vi "Find Unexpected Deps.vi"() -> ()   [LabVIEW 2019, in "DepsWatchToolsMenu.lvlib"]
doc: "GUI to compare LabVIEW code between currently checked out branch with any other branch or any of its commits.\n\n(c) 2024 Soliton Technologies. All rights reserved."
uses:
  DepsWatchToolsMenu.lvlib
  vi.lib/DepsWatch/Typedefs/DepsCheckResult.ctl
  <vilib>/Hampel Software Engineering/Git API/Git API/GIT-api.lvclass
  <vilib>/Hampel Software Engineering/Git API/Git API/GIT-api.lvclass/GIT-api.ctl
  <vilib>/Hampel Software Engineering/Git API/Git API/Controls/GIT-Repository States.ctl
  <vilib>/Hampel Software Engineering/Git API/Git API/Accessors/GIT-Set Working Dir.vi
  <userlib>/_OpenG.lib/file/file.llb/Valid Path - Traditional__ogtk.vi
  <userlib>/_OpenG.lib/file/file.llb/File Exists - Scalar__ogtk.vi
  vi.lib/DepsWatch/DepsWatch.lvlib
panel:
  in  "Tab Control":T1(tab)=enum."Main UI"
  in  "Check Changed Libraries Only?":bool
  out "Unexpected / Missing Deps":T2[](array[typedef])
  in  "Branch to Compare":string(combo)="origin/main"
  in  "Refresh Current Branch":bool
  out "Current Branch":string="origin/main" caption="Current Compare"
  out "Current Branch Status":string
  in  "Stop":bool
  in  "Repository Path":path
  in  "Compare":bool
  # "1. Checkout the branch of interest in your system using any method - Git command line, Desktop Git GUI Clients etc.,\n\n2. Specify the local Repository Path.\n\n3. Verify the current branch, its status and select a branch or commit based on the Compare Mode and click on Compare to display the file changes.\n\n4. Double click on a file to initiate LabVIEW code comparison.\n\n5. Once done with required comparisons, exit the tool by closing the window. The tool cleans up the temporary files added during comparison.\n\n\nNote:\n1. This tool uses LabVIEW's VI Comparison Tool which requires LabVIEW Professional Development System.\n2. It is recommended to not use other Git Clients actively when comparing files using this tool to avoid Git command related errors.\n3. It is recommended to commit all changes (working copy) before using this tool for comparison."
  # "This tool uses git diff command to identify the changes. Hence it is recommended to commit all the changes (working copy) to have them considered for comparison. For code comparison, this tool uses LabVIEW's built in VI Comparison Tool.\n\nExample: Identify changes in current branch when comparing with other branch\n\n---A---B---C---D    <== other branch\n               \\\n                 E---F      <== current branch\n\n1. We will need to identify only the file changes introduced by current branch. E and F commits are those changes in the above example (commits after the common ancestor B).\n2. For the identified file changes compare with the other branch (D) to see how it differs. These differences will be our current branch changelist.\n\nWhy only current branch changes?\nIt is most useful to see how the current branch will modify the files when it is getting merged. Best use case for displaying only current branch changelist will be for Pull Request reviews."
  # "1. Repository Path - Local repository path (the top level folder with '.git' hidden folder in it). Git API will be initialized for this repository.\n\n2. Current Branch - Currently checked out branch. The status of the current branch is also displayed at top right. Click Refresh button to update the current branch if it is changed in the system or received new changes via Git Pull.\n\n3. Compare Mode - Select the type of comparison. You can compare the current branch with another branch or with a particular commit of a selected branch.\n\nIn branch comparison mode, you can enter the branch name for comparison in Branch to Compare. Remote branches usually start with \"origin/\" and local branches do not have \"origin/\" prefix. The branch's recent commit is displayed in Recent Commit and its details in Commit Details for reference. \n\nIn commit comparison mode, the commits available in the branch selected in Select Branch are listed in Commit to Compare. For the commit selected in Commit to Compare, its details will be displayed in the Commit Details. Use Commits to Fetch to limit the number of commits obtained and improve the loading time.\n\n     Note: Git doesn't maintain information on when the branch is created. So, all the commits of the selected branch will be displayed (all the way up to the very first commit after repository creation). Without a limit, it increases loading time.\n\n4. Compare - Identifies the file changes and Current Branch Changelist table shows the list of all files that are different in the current branch compared to the branch/commit selected.\n\n     Note: The other branch/commit in comparison would have introduced its own changes that are not part of current branch. Those changes will not be displayed.\n\n5. Filter LabVIEW VI and Control Files - Filter files except VI and CTL files. These require LabVIEW to compare but project, library and classes are text files that can be easily reviewed in the desktop Git GUI clients or in Pull Request of Git web services.\n\n6. LabVIEW Compare Options - Options to decide what to compare in the code. Set the required options before initiating code compare.\n\n7. Double click on the file you wish to compare. LabVIEW opens the compare window for the file from the current branch and the file from the other branch/commit (file will be suffixed with TEMP). It may take a while if the VI/CTL have lot of dependencies to load. Having the project pre-opened and opening this tool from that instance may reduce the loading time. Note that the file from the other branch/commit in comparison may be missing its dependent files which may not be available in the current branch or deleted in the current branch commits. This will cause the file to be in a broken state but does not affect the comparison. Another reason for the broken state may be due to the parent library/class not recognizing this new file with the suffix but this as well will not affect the comparison.\n\n     Note: The files from other branch/commit are placed at the same location in the current branch so that the LabVIEW can load the dependencies appropriately.\n\n8. Viewed Status (mixed checkbox) - A tick mark appears for every file compared or opened. Use the mixed checkbox (below the Current Branch Changelist) to control status for all files.\n\n     Note: Viewed status is only a visual aid for tracking and does not have any other function other than that.\n\n9. Panel Close - Stops the tools execution after removing all the new files introduced into the current branch (TEMP files)."
  # "This GUI helps identify unexpected dependencies across all libraries in a repository. It also supports branch-to-branch comparison, allowing users to analyze dependency changes between any two branches and validate dependencies only for the modified libraries."
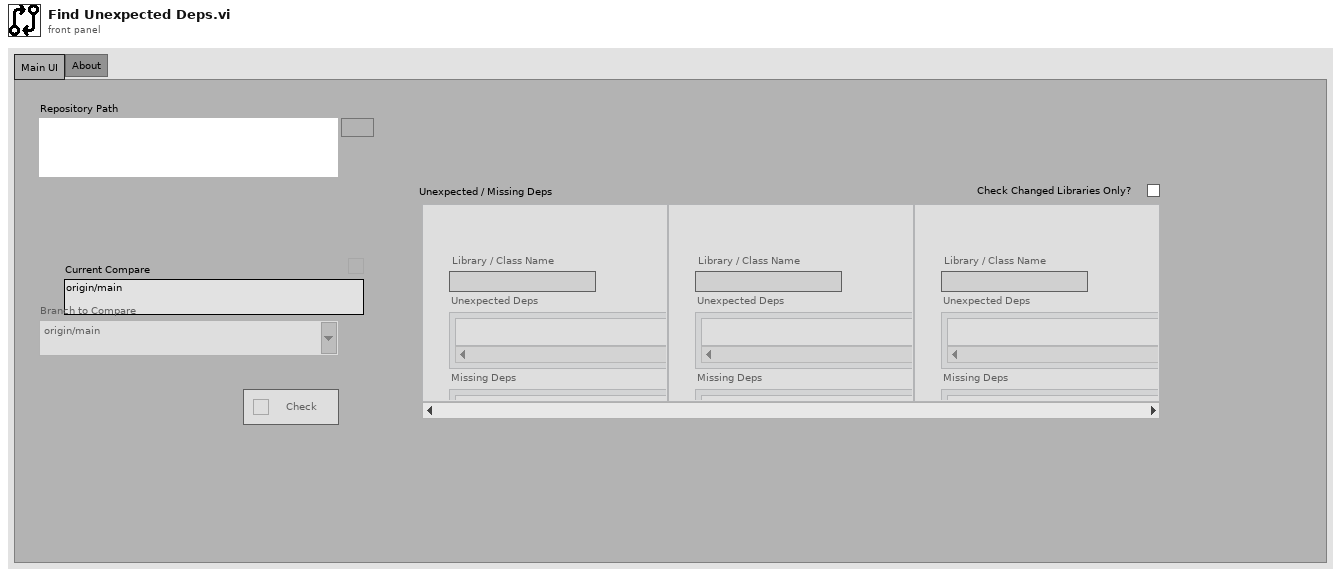
[diagram p1: front panel]
types:
  T1 = enum32{"Getting Started", "How it Works?", "Main UI", "Help", "About"}
  T2 = typedef "DepsWatch.lvlib/DepsCheckResult.ctl" = cluster{"Library / Class Name":string, "Unexpected Deps":cluster{"Dependency":string, "IsDirect?":bool}[], "Missing Deps":cluster{"Dependency":string, "IsDirect?":bool}[]}
  T3 = cluster{"Repository Path":path, "Git API Object":refnum<class "GIT-api.lvclass">, "Git API Initialized?":bool, "Current Branch":string, "Branch to Compare":string, "Check Changed Libraries Only?":bool, "Failures":T2[]}
  T4 = typedef "GIT-API-for-LabVIEW.lvlib/GIT-api.lvclass/GIT-Repository States.ctl" = enum16{"up-to-date", "behind", "ahead", "diverged", "unpublished", "detached", "unknown"}
  T5 = enum8{"Enabled", "Disabled", "Disabled and Grayed Out"}
  T6 = typedef "DepsWatch.lvlib/CICDPathConfigs.ctl" = cluster{"GlobalIncludePaths":path[], "GlobalExcludePaths":path[], "BuildSpecsIncludePaths":path[], "ActualDepsIncludePaths":path[], "WorkspacePath":path, "SourceFolderPaths":path[], "ChangedFilesLogpaths":map{string, path}}
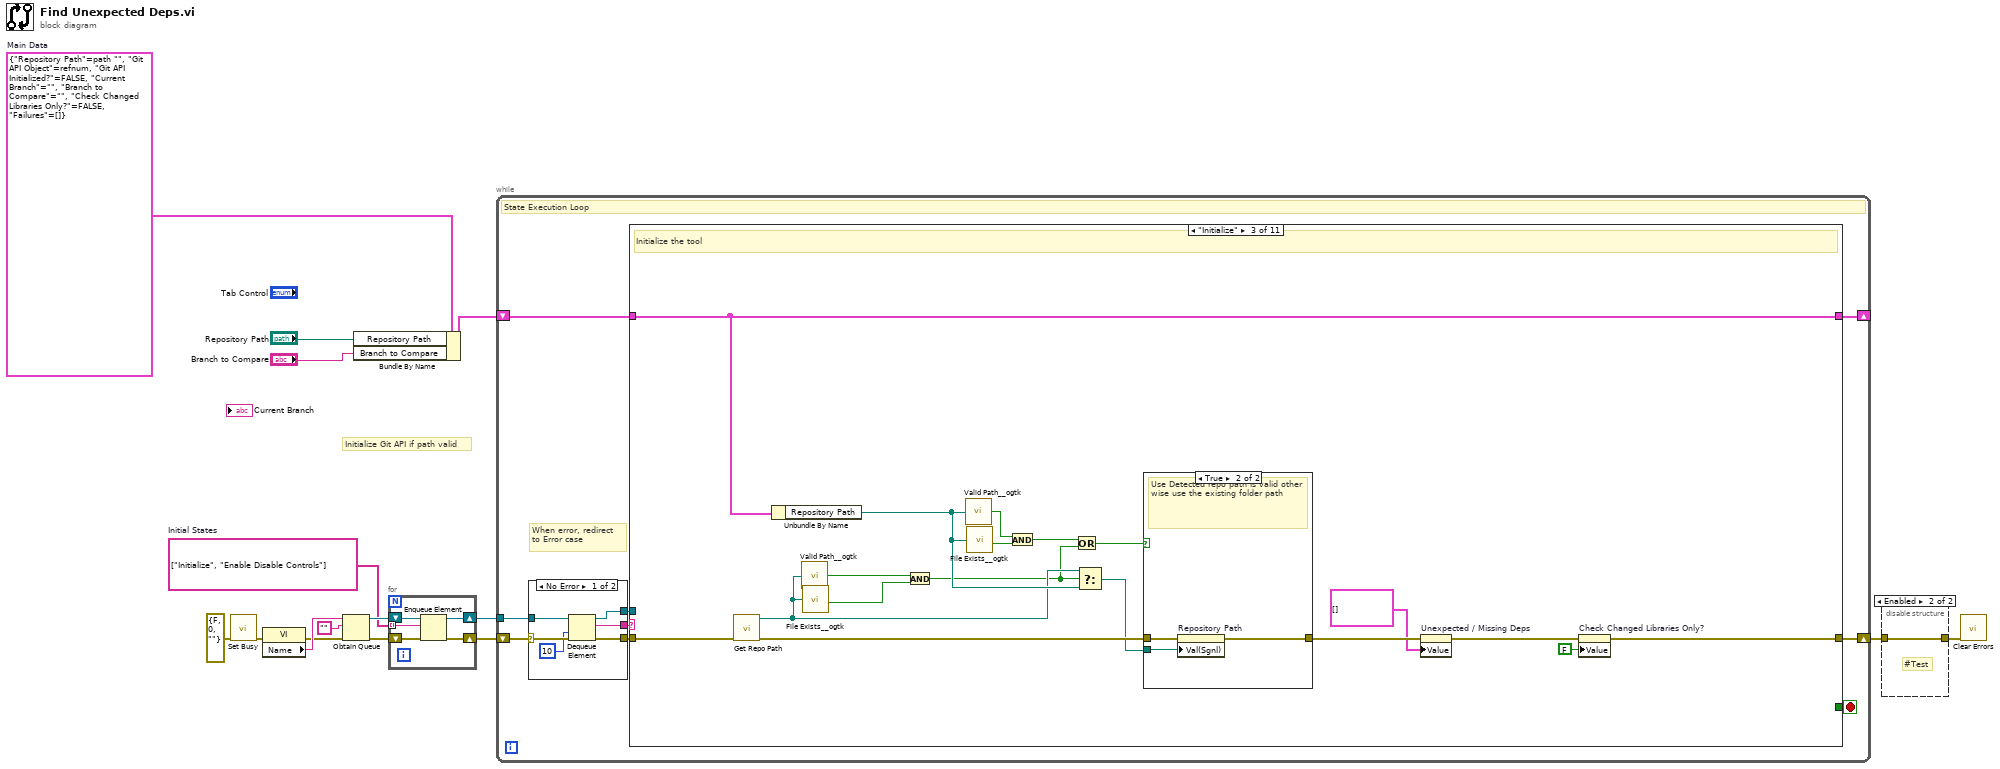
[diagram p0: block diagram]
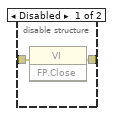
[diagram p2: hidden frame]
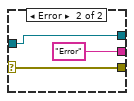
[diagram p3: hidden frame]
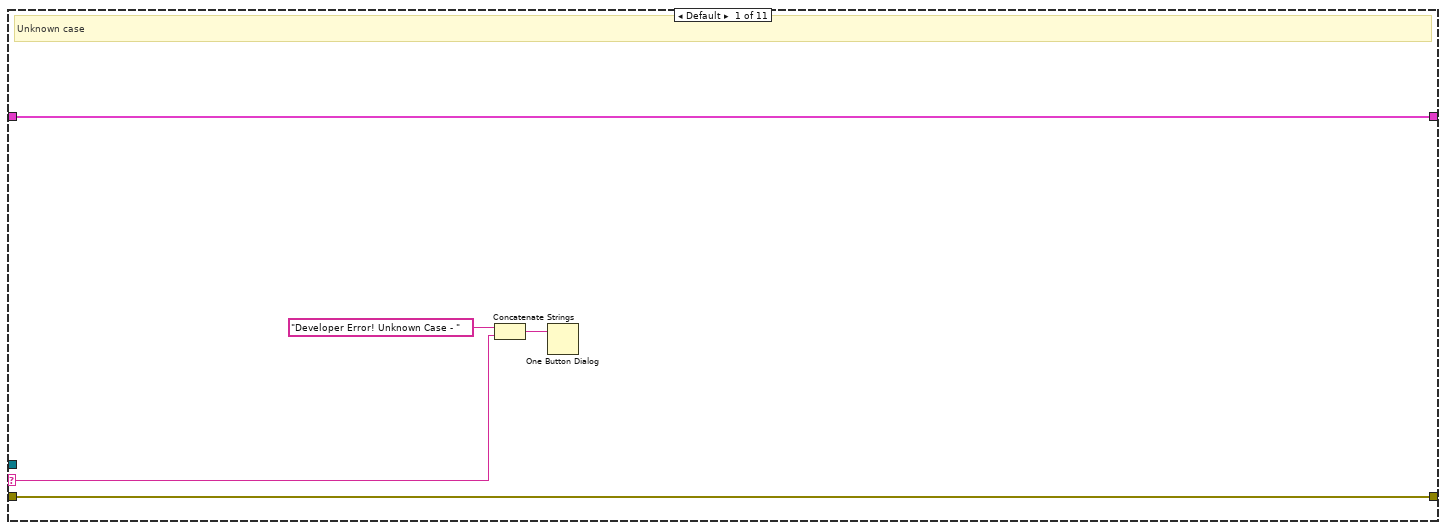
[diagram p4: hidden frame]
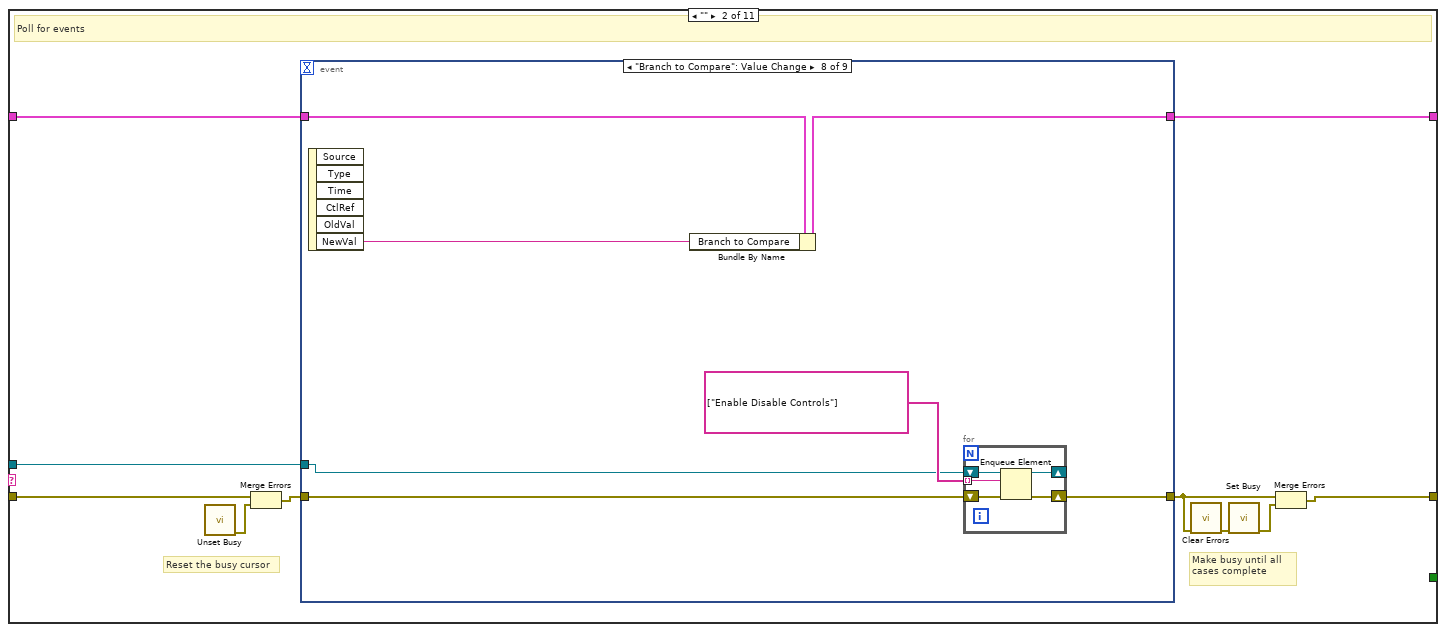
[diagram p5: hidden frame]
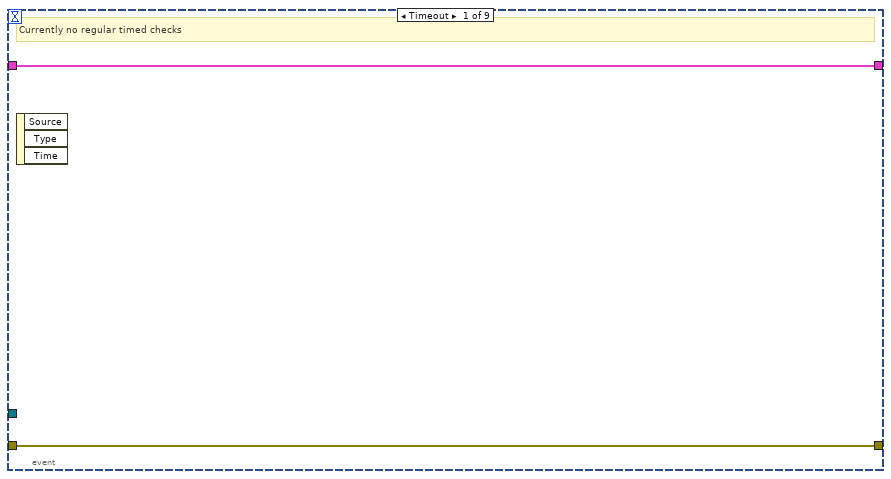
[diagram p6: hidden frame]
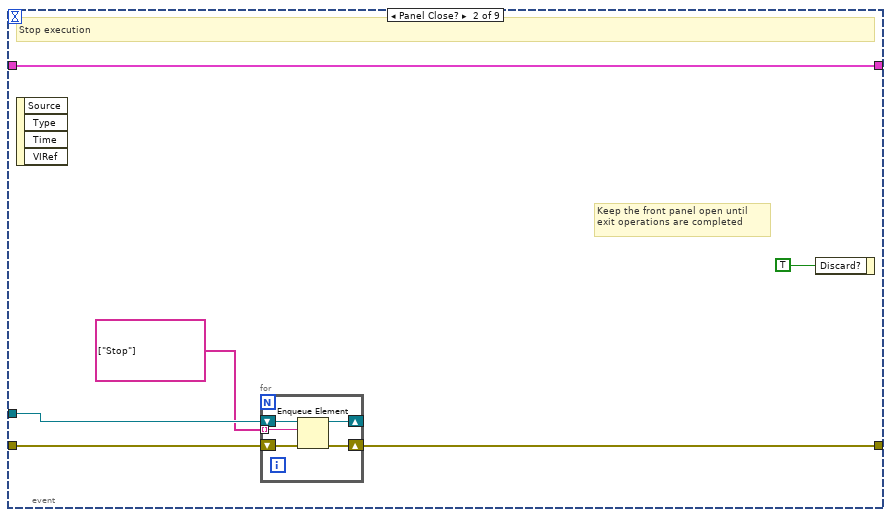
[diagram p7: hidden frame]
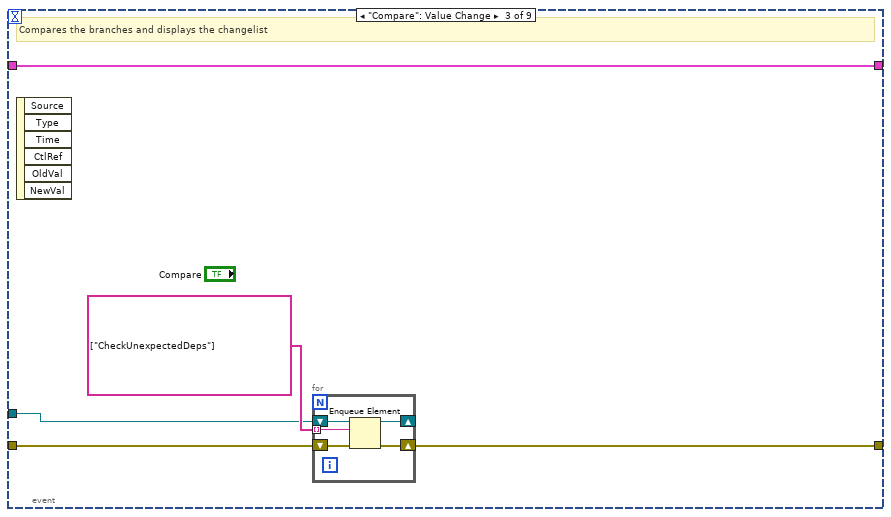
[diagram p8: hidden frame]
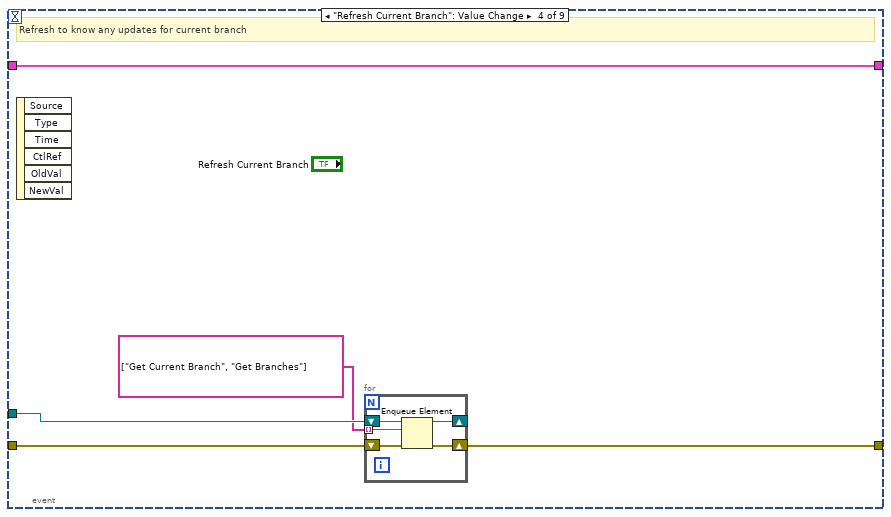
[diagram p9: hidden frame]
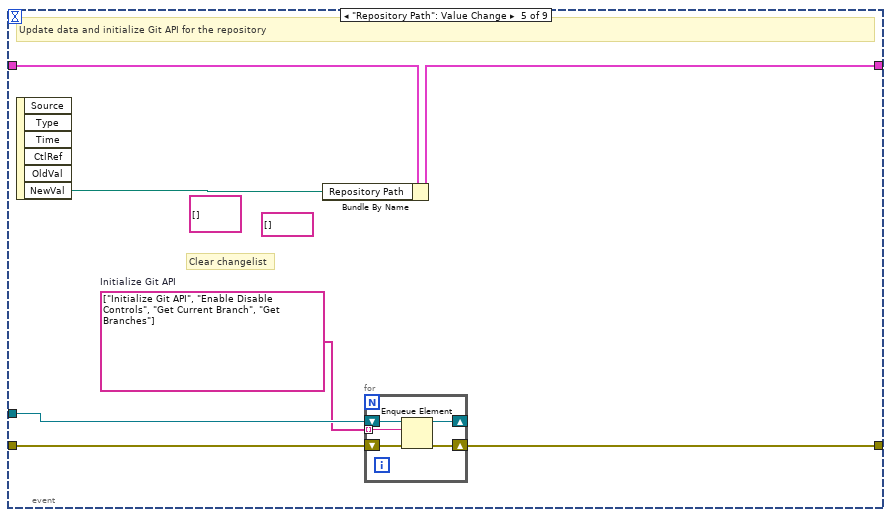
[diagram p10: hidden frame]
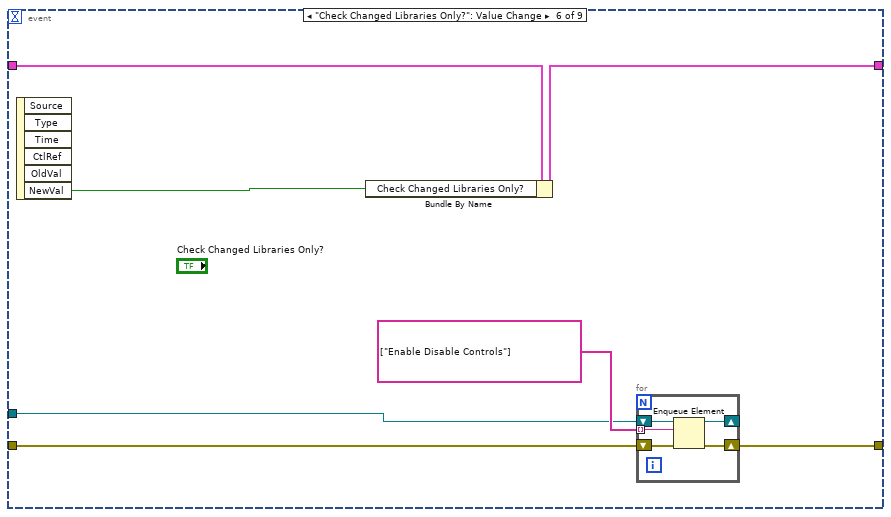
[diagram p11: hidden frame]
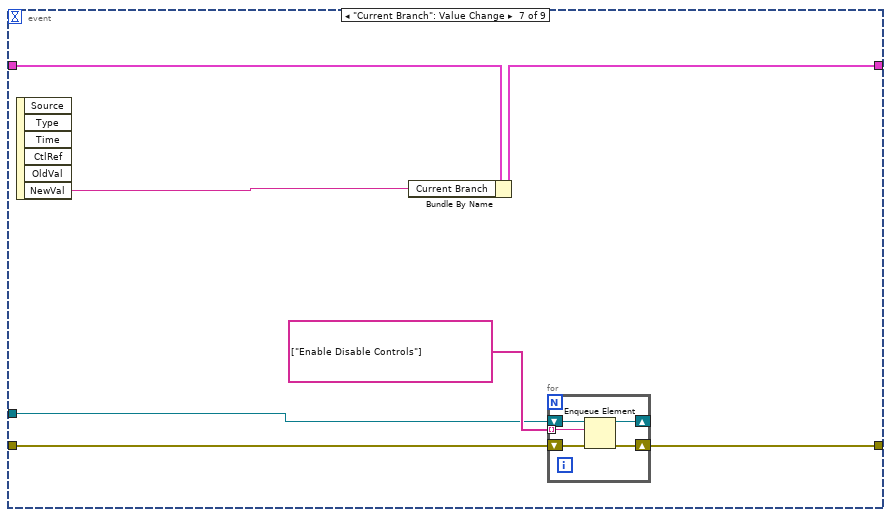
[diagram p12: hidden frame]
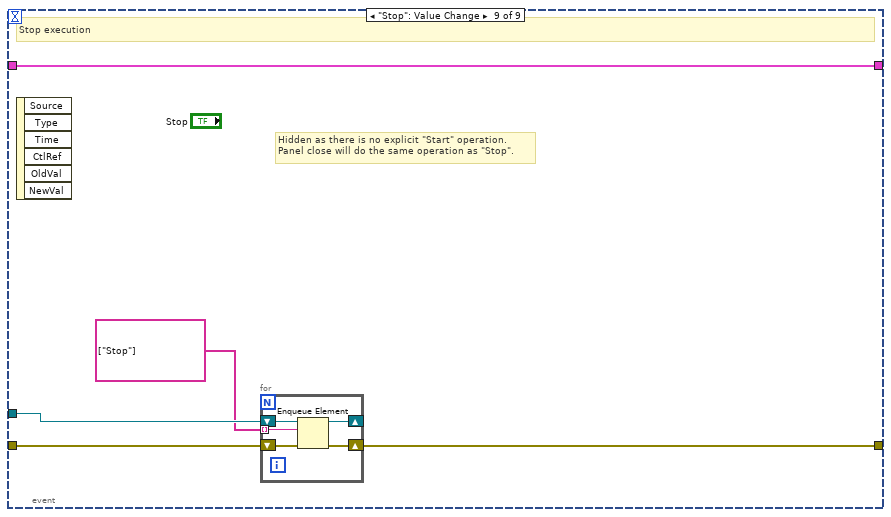
[diagram p13: hidden frame]
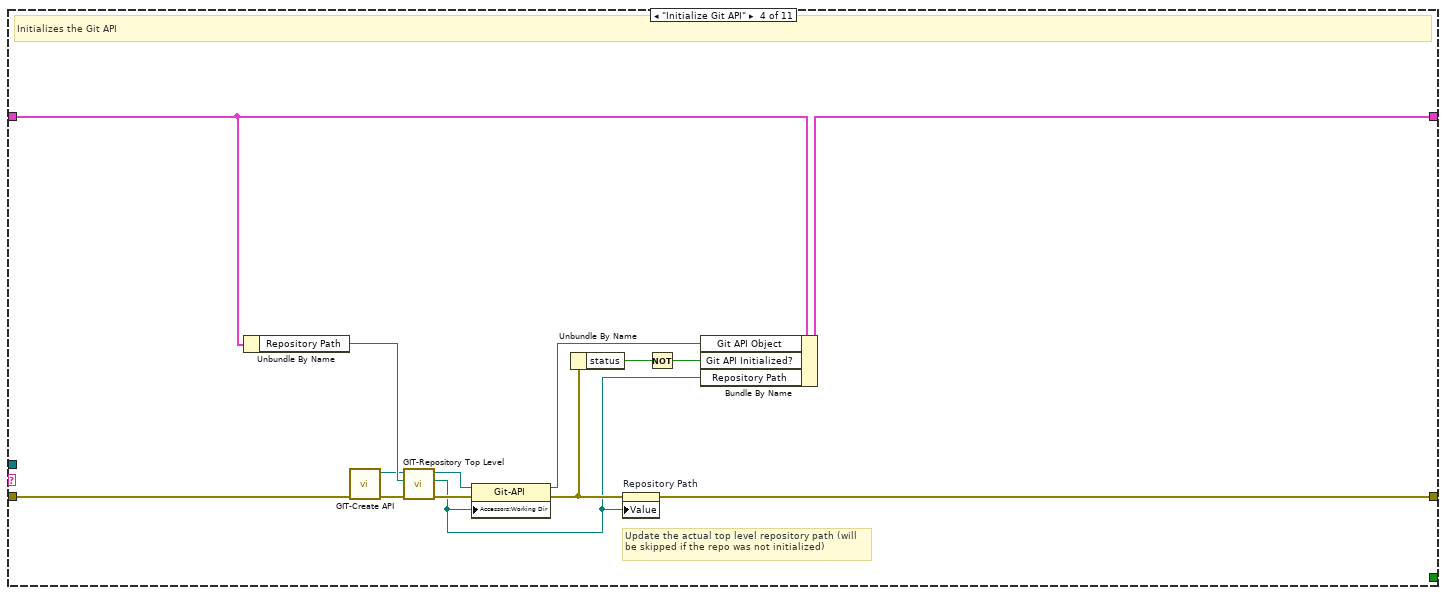
[diagram p15: hidden frame]
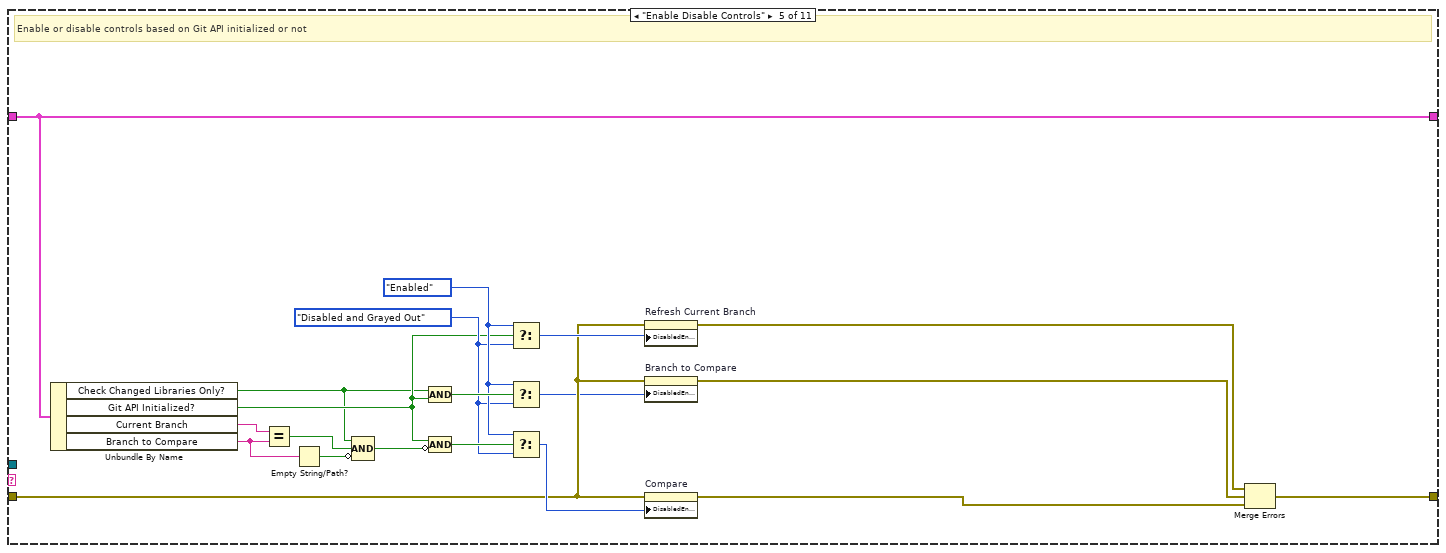
[diagram p16: hidden frame]
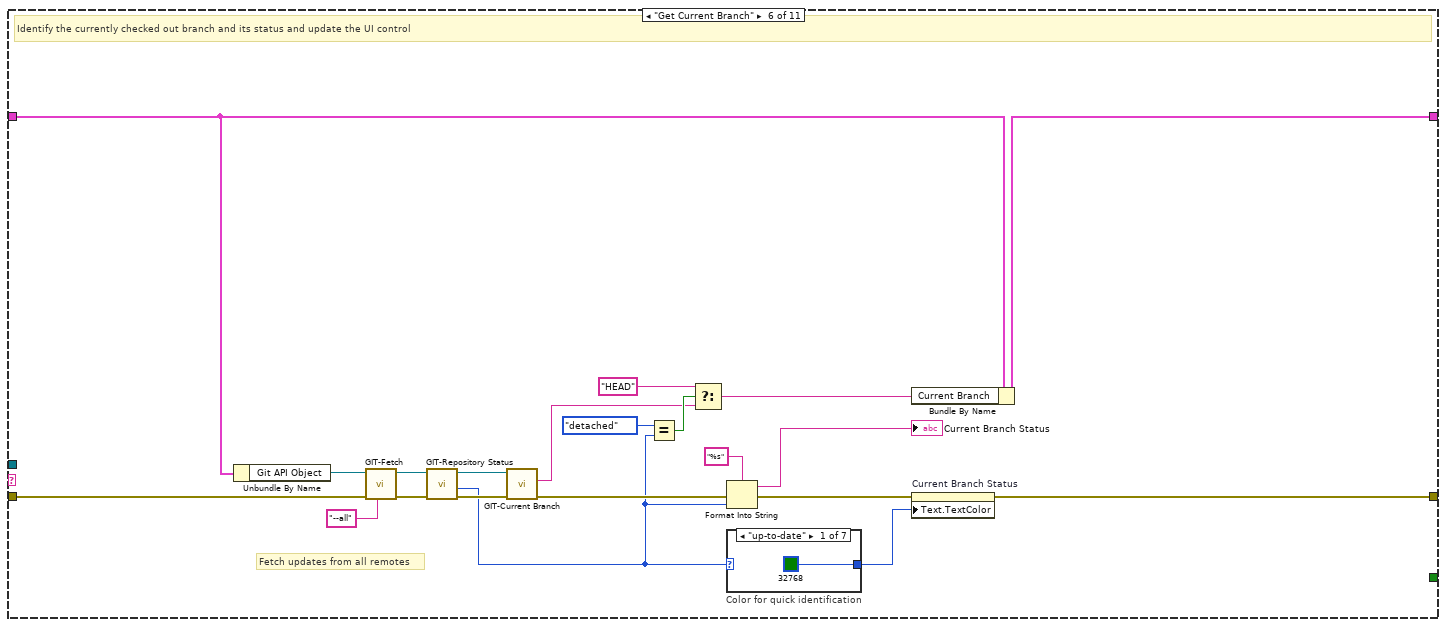
[diagram p17: hidden frame]
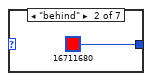
[diagram p18: hidden frame]
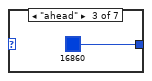
[diagram p19: hidden frame]
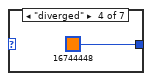
[diagram p20: hidden frame]
diagram:
  w1 = string[] ["Initialize", "Enable Disable Controls"]  # Initial States
  w13 = T3 {"Repository Path"=path "", "Git API Object"=refnum, "Git API Initialized?"=FALSE, "Current Branch"="", "Branch to Compare"="", "Check Changed Libraries Only?"=FALSE, "Failures"=[]}  # Main Data
  # "Initialize Git API if path valid"
  n1 = call <vilib>:"Set Busy.vi"("error in (no error)"=errorcluster {"status"=FALSE, "code"=0, "source"=""}) -> ("error out"=w6:errorcluster)  [unwired: 9 in, 1 out]
  n2 = property class="VI"(error in=w6) -> (error out=w15:errorcluster, "Name"=w16:string)  [unwired: 1 in, 1 out]
  n3 = Obtain Queue(name (unnamed)=w16, element data type="", error in (no error)=w15) -> (queue out=w11:refnum<queue>, error out=w8:errorcluster)  [unwired: 2 in, 1 out]
  n4 = Bundle By Name(cluster=w13, "Repository Path"="Repository Path", "Branch to Compare"="Branch to Compare") -> (w12:T3)
  n5 = for {
    tunnel: w1 -> [w18] mode=indexing
    shift-right: [w20] -> w10
    shift-left: w8 -> [w21]
    shift-right: [w17] -> w9
    shift-left: w11 -> [w19]
    n6 = Enqueue Element(queue=w19, element=w18, error in (no error)=w21) -> (queue out=w17:refnum<queue>, error out=w20:errorcluster)  [unwired: 1 in, 1 out]
  }
  n7 = while {
    shift-right: [w22] -> w4
    shift-left: w10 -> [w24]
    tunnel: w9 -> [w25]
    shift-right: [w27] -> _
    shift-left: w12 -> [w26]
    stop <- w28 stop-if-true
    # "When error, redirect to Error case"
    # "State Execution Loop"
    n8 = case shown="No Error" w24 {
      selector: w24 -> [w33 w37]
      tunnel: [w36 "Error" ("element")] -> w30
      tunnel: [w35 w39] -> w29
      tunnel: w25 -> [w34 w39]
      tunnel: [w31 w37] -> w23
      frame No Error {
        n9 = Dequeue Element(queue=w34, timeout in ms (-1)=10, error in (no error)=w33) -> (queue out=w35:refnum<queue>, element=w36:string, error out=w31:errorcluster)  [unwired: 1 out]
      }
      frame Error {
      }
    }
    n10 = case shown="\"Initialize\"" w30 {
      selector: w30 -> [w43 _ _ _ _ _ _ _ _ _ _]
      tunnel: w23 -> [w41 w48 w160 w181 w193 w207 w234 w277 w301 w311 w319]
      tunnel: w29 -> [_ w54 _ _ _ _ _ _ w299 w308 w316]
      tunnel: [w41 w50 w163 w169 w199 w216 w235 w286 w300 w307 w312] -> w22
      tunnel: [_ _ _ _ _ _ _ _ _ w309 _] -> w28
      tunnel: [w40 w52 w154 w178 w201 w219 w233 w284 w298 w310 w320] -> w27
      tunnel: w26 -> [w40 w53 w154 w180 w201 w220 w238 w285 w298 w310 w320]
      frame Default {
        # "Unknown case"
        n11 = Concatenate Strings("Developer Error! Unknown Case - " ("string"), w43) -> (w42:string)
        n12 = One Button Dialog(message=w42) -> ()  [unwired: 1 in, 1 out]
      }
      frame "" {
        # "Reset the busy cursor"
        # "Make busy until all cases complete"
        # "Poll for events"
        n13 = call <vilib>:"Unset Busy.vi"() -> ("error out"=w49:errorcluster)  [unwired: 11 in]
        n14 = Merge Errors(w48, w49) -> (w47:errorcluster)
        n15 = event shown="[7] \"Branch to Compare\": Value Change" {
          selector: _ -> [_ _ _ _ _ _ _ _ _]
          dyn-events: _ -> [_ _ _ _ _ _ _ _ _]
          timeout: _ -> [_ _ _ _ _ _ _ _ _]
          tunnel: w47 -> [w55 w62 w71 w82 w91 w101 w112 w124 w140]
          tunnel: w54 -> [_ w61 w70 w81 w90 w100 w114 w126 w139]
          tunnel: [w55 w60 w69 w79 w89 w102 w113 w125 w138] -> w46
          tunnel: w53 -> [w56 w59 w68 w78 w94 w106 w118 w130 w137]
          tunnel: [w56 w59 w68 w78 w93 w105 w117 w129 w137] -> w52
          event Timeout {
            # "Currently no regular timed checks"
            n16 = event-data() -> ()  [unwired: 1 in, 3 out]
          }
          event Panel Close? {
            # "Keep the front panel open until exit operations are completed"
            # "Stop execution"
            n17 = event-data() -> ()  [unwired: 1 in, 4 out]
            n18 = for {
              tunnel: string[] ["Stop"] -> [w64] mode=indexing
              shift-right: [w66] -> w60
              shift-left: w62 -> [w67]
              shift-right: [w63] -> _
              shift-left: w61 -> [w65]
              n19 = Enqueue Element(queue=w65, element=w64, error in (no error)=w67) -> (queue out=w63:refnum<queue>, error out=w66:errorcluster)  [unwired: 1 in, 1 out]
            }
            n20 = event-data("Discard?"=TRUE) -> ()  [unwired: 1 in, 1 out]
          }
          event "Compare": Value Change {
            # "Compares the branches and displays the changelist"
            n21 = event-data() -> ()  [unwired: 1 in, 6 out]
            n22 = for {
              tunnel: string[] ["CheckUnexpectedDeps"] -> [w74] mode=indexing
              shift-right: [w76] -> w69
              shift-left: w71 -> [w77]
              shift-right: [w73] -> _
              shift-left: w70 -> [w75]
              n23 = Enqueue Element(queue=w75, element=w74, error in (no error)=w77) -> (queue out=w73:refnum<queue>, error out=w76:errorcluster)  [unwired: 1 in, 1 out]
            }
          }
          event "Refresh Current Branch": Value Change {
            # "Refresh to know any updates for current branch"
            n24 = event-data() -> ()  [unwired: 1 in, 6 out]
            n25 = for {
              tunnel: string[] ["Get Current Branch", "Get Branches"] -> [w84] mode=indexing
              shift-right: [w86] -> w79
              shift-left: w82 -> [w87]
              shift-right: [w83] -> _
              shift-left: w81 -> [w85]
              n26 = Enqueue Element(queue=w85, element=w84, error in (no error)=w87) -> (queue out=w83:refnum<queue>, error out=w86:errorcluster)  [unwired: 1 in, 1 out]
            }
          }
          event "Repository Path": Value Change {
            w88 = string[] ["Initialize Git API", "Enable Disable Controls", "Get Current Branch", "Get Branches"]  # Initialize Git API
            (unwired) string[] [] ("Viewed Files")
            (unwired) string[][] [] ("Item Names")
            # "Clear changelist"
            # "Update data and initialize Git API for the repository"
            n27 = event-data() -> ("NewVal"=w92:path)  [unwired: 1 in, 5 out]
            n28 = Bundle By Name(cluster=w94, "Repository Path"=w92) -> (w93:T3)
            n29 = for {
              tunnel: w88 -> [w96] mode=indexing
              shift-right: [w98] -> w89
              shift-left: w91 -> [w99]
              shift-right: [w95] -> _
              shift-left: w90 -> [w97]
              n30 = Enqueue Element(queue=w97, element=w96, error in (no error)=w99) -> (queue out=w95:refnum<queue>, error out=w98:errorcluster)  [unwired: 1 in, 1 out]
            }
          }
          event "Check Changed Libraries Only?": Value Change {
            n31 = event-data() -> ("NewVal"=w104:bool)  [unwired: 1 in, 5 out]
            n32 = Bundle By Name(cluster=w106, "Check Changed Libraries Only?"=w104) -> (w105:T3)
            n33 = for {
              tunnel: string[] ["Enable Disable Controls"] -> [w108] mode=indexing
              shift-right: [w110] -> w102
              shift-left: w101 -> [w111]
              shift-right: [w107] -> _
              shift-left: w100 -> [w109]
              n34 = Enqueue Element(queue=w109, element=w108, error in (no error)=w111) -> (queue out=w107:refnum<queue>, error out=w110:errorcluster)  [unwired: 1 in, 1 out]
            }
          }
          event "Current Branch": Value Change {
            n35 = event-data() -> ("NewVal"=w116:string)  [unwired: 1 in, 5 out]
            n36 = Bundle By Name(cluster=w118, "Current Branch"=w116) -> (w117:T3)
            n37 = for {
              tunnel: string[] ["Enable Disable Controls"] -> [w120] mode=indexing
              shift-right: [w122] -> w113
              shift-left: w112 -> [w123]
              shift-right: [w119] -> _
              shift-left: w114 -> [w121]
              n38 = Enqueue Element(queue=w121, element=w120, error in (no error)=w123) -> (queue out=w119:refnum<queue>, error out=w122:errorcluster)  [unwired: 1 in, 1 out]
            }
          }
          event "Branch to Compare": Value Change {
            n39 = event-data() -> ("NewVal"=w128:string)  [unwired: 1 in, 5 out]
            n40 = Bundle By Name(cluster=w130, "Branch to Compare"=w128) -> (w129:T3)
            n41 = for {
              tunnel: string[] ["Enable Disable Controls"] -> [w132] mode=indexing
              shift-right: [w134] -> w125
              shift-left: w124 -> [w135]
              shift-right: [w131] -> _
              shift-left: w126 -> [w133]
              n42 = Enqueue Element(queue=w133, element=w132, error in (no error)=w135) -> (queue out=w131:refnum<queue>, error out=w134:errorcluster)  [unwired: 1 in, 1 out]
            }
          }
          event "Stop": Value Change {
            # "Hidden as there is no explicit \"Start\" operation.\nPanel close will do the same operation as \"Stop\"."
            # "Stop execution"
            n43 = event-data() -> ()  [unwired: 1 in, 6 out]
            n44 = for {
              tunnel: string[] ["Stop"] -> [w142] mode=indexing
              shift-right: [w144] -> w138
              shift-left: w140 -> [w145]
              shift-right: [w141] -> _
              shift-left: w139 -> [w143]
              n45 = Enqueue Element(queue=w143, element=w142, error in (no error)=w145) -> (queue out=w141:refnum<queue>, error out=w144:errorcluster)  [unwired: 1 in, 1 out]
            }
          }
        }
        n46 = call <vilib>:"Clear Errors.vi"("error in (no error)"=w46) -> ("error out"=w45:errorcluster)  [unwired: 5 in, 1 out]
        n47 = call <vilib>:"Set Busy.vi"("error in (no error)"=w45) -> ("error out"=w51:errorcluster)  [unwired: 9 in, 1 out]
        n48 = Merge Errors(w46, w51) -> (w50:errorcluster)
      }
      frame "Initialize" {
        # "Initialize the tool"
        n49 = call "Get Repo Path.vi"("error in (no error)"=w160) -> ("error out"=w161:errorcluster, "Repo Path"=w148:path)  [unwired: 9 in]
        n50 = Unbundle By Name(w154) -> ("Repository Path"=w150:path)
        n51 = call-poly <userlib>:"Valid Path__ogtk.vi"("path"=w148) -> ("valid"=w157:bool)
        n52 = call-poly <userlib>:"File Exists__ogtk.vi"("file path"=w148) -> ("exists"=w158:bool)  [unwired: 6 in, 1 out]
        n53 = And(x=w157, y=w158) -> (x .and. y?=w146:bool)
        n54 = call-poly <userlib>:"Valid Path__ogtk.vi"("path"=w150) -> ("valid"=w149:bool)
        n55 = call-poly <userlib>:"File Exists__ogtk.vi"("file path"=w150) -> ("exists"=w153:bool)  [unwired: 6 in, 1 out]
        n56 = And(x=w149, y=w153) -> (x .and. y?=w152:bool)
        n57 = Or(x=w152, y=w146) -> (x .or. y?=w151:bool)
        n58 = Select(t=w148, s=w146, f=w150) -> (s? t:f=w147:path)
        n59 = case shown="True" w151 {
          tunnel: w161 -> [w164 w167]
          tunnel: [w164 w165] -> w159
          tunnel: w147 -> [_ w166]
          frame False {
          }
          frame True {
            # "Use Detected repo path is valid other wise use the existing folder path"
            n60 = property on="Repository Path" class="Path"(error in=w167, "Val(Sgnl)"=w166) -> (error out=w165:errorcluster)  [unwired: 1 in, 1 out]
          }
        }
        n61 = property on="Unexpected / Missing Deps" class="Arr (strict)"(error in=w159, "Value"=T2[] [] ("Unexpected / Missing Deps")) -> (error out=w156:errorcluster)  [unwired: 1 in, 1 out]
        n62 = property on="Check Changed Libraries Only?" class="Bool (strict)"(error in=w156, "Value"=FALSE ("Check Changed Libraries Only?")) -> (error out=w163:errorcluster)  [unwired: 1 in, 1 out]
      }
      frame "Initialize Git API" {
        # "Update the actual top level repository path (will be skipped if the repo was not initialized)"
        # "Initializes the Git API"
        n63 = Unbundle By Name(w180) -> ("Repository Path"=w177:path)
        n64 = call <vilib>:"GIT-Create API.vi"("error in"=w181) -> ("error out"=w176:errorcluster, "git-api out"=w174:refnum<class "GIT-api.lvclass">)  [unwired: 9 in]
        n65 = call <vilib>:"GIT-Repository Top Level.vi"("error in"=w176, "Current Path"=w177, "git-api in"=w174) -> ("error out"=w173:errorcluster, "Repo Top Level Path"=w168:path, "git-api out"=w175:refnum<class "GIT-api.lvclass">)  [unwired: 6 in]
        n66 = property class="Git-API"(reference=w175, error in=w173, "Accessors:Working Dir"=w168) -> (reference out=w179:refnum<class "GIT-api.lvclass">, error out=w170:errorcluster)
        n67 = Unbundle By Name(w170) -> ("status"=w172:bool)
        n68 = property on="Repository Path" class="Path"(error in=w170, "Value"=w168) -> (error out=w169:errorcluster)  [unwired: 1 in, 1 out]
        n69 = Not(x=w172) -> (.not. x?=w171:bool)
        n70 = Bundle By Name(cluster=w180, "Git API Object"=w179, "Git API Initialized?"=w171, "Repository Path"=w168) -> (w178:T3)
      }
      frame "Enable Disable Controls" {
        w189 = T5."Disabled and Grayed Out" ("Disabled")
        w191 = T5."Enabled" ("Disabled")
        # "Enable or disable controls based on Git API initialized or not"
        n71 = Unbundle By Name(w201) -> ("Check Changed Libraries Only?"=w182:bool, "Git API Initialized?"=w184:bool, "Current Branch"=w195:string, "Branch to Compare"=w187:string)
        n72 = Equal?(x=w195, y=w187) -> (x = y?=w183:bool)
        n73 = Empty String/Path?(string/path=w187) -> (empty?=w186:bool)
        n74 = Compound Arithmetic op=AND(w182, w183, invert w186) -> (w185:bool)
        n75 = Compound Arithmetic op=AND(w182, w184) -> (w192:bool)
        n76 = Compound Arithmetic op=AND(w184, invert w185) -> (w196:bool)
        n77 = Select(t=w191, s=w184, f=w189) -> (s? t:f=w194:T5)
        n78 = Select(t=w191, s=w192, f=w189) -> (s? t:f=w190:T5)
        n79 = Select(t=w191, s=w196, f=w189) -> (s? t:f=w197:T5)
        n80 = property on="Refresh Current Branch" class="Bool"(error in=w193, "DisabledEnum"=w194) -> (error out=w200:errorcluster)  [unwired: 1 in, 1 out]
        n81 = property on="Branch to Compare" class="CmbBox"(error in=w193, "DisabledEnum"=w190) -> (error out=w198:errorcluster)  [unwired: 1 in, 1 out]
        n82 = property on="Compare" class="Bool"(error in=w193, "DisabledEnum"=w197) -> (error out=w188:errorcluster)  [unwired: 1 in, 1 out]
        n83 = Merge Errors(w200, w198, w188) -> (w199:errorcluster)
      }
      frame "Get Current Branch" {
        # "Fetch updates from all remotes"
        # "Identify the currently checked out branch and its status and update the UI control"
        n84 = Unbundle By Name(w220) -> ("Git API Object"=w208:refnum<class "GIT-api.lvclass">)
        n85 = call <vilib>:"GIT-Fetch.vi"("param"="--all", "error in"=w207, "git-api in"=w208) -> ("error out"=w213:errorcluster, "git-api out"=w214:refnum<class "GIT-api.lvclass">)  [unwired: 6 in, 1 out]
        n86 = call <vilib>:"GIT-Repository Status.vi"("error in"=w213, "git-api in"=w214) -> ("error out"=w222:errorcluster, "State"=w205:T4, "git-api out"=w221:refnum<class "GIT-api.lvclass">)  [unwired: 6 in, 1 out]
        n87 = call <vilib>:"GIT-Current Branch.vi"("error in"=w222, "git-api in"=w221) -> ("error out"=w206:errorcluster, "current branch"=w209:string)  [unwired: 7 in, 1 out]
        n88 = Equal?(x=GIT-Repository_States."detached", y=w205) -> (x = y?=w210:bool)
        n89 = Select(t="HEAD", s=w210, f=w209) -> (s? t:f=w202:string)
        n90 = Format Into String(format string="%s", error in=w206, w205) -> (resulting string=→"Current Branch Status":string, error out=w203:errorcluster)  [unwired: 1 in]
        n91 = case "Color for quick identification" shown="\"up-to-date\"" w205 {
          tunnel: [u32 32768 u32 16711680 u32 16860 u32 16744448 u32 16777222 u32 7171459 u32 16711680] -> w215
          frame "up-to-date" {
          }
          frame "behind" {
          }
          frame "ahead" {
          }
          frame "diverged" {
          }
          frame "unpublished" {
          }
          frame "detached" {
          }
          frame "unknown" {
          }
        }
        n92 = Bundle By Name(cluster=w220, "Current Branch"=w202) -> (w219:T3)
        n93 = property on="Current Branch Status" class="Str"(error in=w203, "Text.TextColor"=w215) -> (error out=w216:errorcluster)  [unwired: 1 in, 1 out]
      }
      frame "CheckUnexpectedDeps" {
        w240 = TRUE  # GUI Mode? {F)
        n94 = Unbundle By Name(w238) -> ("Repository Path"=w237:path, "Check Changed Libraries Only?"=w236:bool, "Current Branch"=w231:string, "Branch to Compare"=w230:string)
        n95 = case shown="True" w236 {
          tunnel: [w241 w252] -> w239
          tunnel: w240 -> [_ w251]
          tunnel: w237 -> [_ w246]
          tunnel: w234 -> [w241 w245]
          tunnel: w231 -> [_ w243]
          tunnel: w230 -> [_ w242]
          frame False {
          }
          frame True {
            # "Update Changed Libraries List."
            n96 = call "ReadCICDPathConfig.vi"("error in (no error)"=w245, "Workspace Path"=w246) -> ("error out"=w244:errorcluster, "CICD Path Config Out"=w250:T6)  [unwired: 8 in]
            n97 = Unbundle By Name(w250) -> ("ChangedFilesLogpaths"=w248:map{string, path})
            n98 = Look In Map(map=w248, key="InScopeChangedLVFilesPath") -> (value=w247:path)  [unwired: 1 in, 1 out]
            n99 = call "GenerateChangedFilesList.vi"("GUI Mode? {F)"=w251, "Output File Path"=w247, "error in (no error)"=w244, "Branch 2"=w242, "Branch 1"=w243, "Workspace Path"=w246) -> ("error out"=w253:errorcluster)  [unwired: 5 in]
            n100 = call "GenerateChangedLibrariesList.vi"("GUI Mode? {F)"=w251, "error in (no error)"=w253, "Workspace Path"=w246) -> ("error out"=w252:errorcluster)  [unwired: 8 in]
          }
        }
        n101 = call "UnexpectedDepsCheck.vi"("GUI Mode? {F)"=w240, "error in (no error)"=w239, "CheckChangedLibrariesOnly"=w236, "Workspace Path"=w237) -> ("error out"=w235:errorcluster, "Failures"=w232:T2[])  [unwired: 5 in, 1 out]
        "Unexpected / Missing Deps" <- w232
        n102 = Bundle By Name(cluster=w238, "Failures"=w232) -> (w233:T3)
      }
      frame "Get Branches" {
        w267 = 0  # Branch Name List
        w272 = string[][] []
        w271 = "%s" ("format string")
        # "Reset if previous value not found"
        # "Combine local and remote branches"
        # "List Local branches"
        # "List Remote branches\nNote: All remote branches usually start with origin/ unless renamed"
        # "Reset if previous value not found"
        # "Get all local and remote branches and update UI control"
        n103 = Unbundle By Name(w285) -> ("Current Branch"=w257:string, "Git API Object"=w275:refnum<class "GIT-api.lvclass">)
        n104 = call <vilib>:"GIT-Branch.vi"("error in"=w277, "git-api in"=w275) -> ("error out"=w276:errorcluster, "std out"=w268:string, "git-api out"=w269:refnum<class "GIT-api.lvclass">)  [unwired: 7 in]
        n105 = call <vilib>:"GIT-Branch.vi"("param"="-r", "error in"=w276, "git-api in"=w269) -> ("error out"=w279:errorcluster, "std out"=w270:string)  [unwired: 6 in, 1 out]
        n106 = Spreadsheet String To Array(format string=w271, spreadsheet string=w268, array type (2D Dbl)=w272) -> (array=w287:string[][])  [unwired: 1 in]
        n107 = Spreadsheet String To Array(format string=w271, spreadsheet string=w270, array type (2D Dbl)=w272) -> (array=w273:string[][])  [unwired: 1 in]
        n108 = Index Array(array=w287, index (col)=w267) -> (element=w274:string[])  [unwired: 1 in]
        n109 = Index Array(array=w273, index (col)=w267) -> (element=w263:string[])  [unwired: 1 in]
        n110 = for "Remove current branch pointer" {
          tunnel: w274 -> [w296] mode=indexing
          tunnel: [w292] -> w266 mode=indexing
          tunnel: [w291] -> w288 mode=indexing
          n111 = Search and Replace String(input string=w296, search string="*", replace string="") -> (result string=w293:string, error out=w291:errorcluster)  [unwired: 5 in, 2 out]
          n112 = call <vilib>:"Trim Whitespace.vi"("string"=w293) -> ("trimmed string"=w292:string)  [unwired: 1 in]
        }
        n113 = for {
          tunnel: [w290] -> w264 mode=indexing
          tunnel: w263 -> [w289] mode=indexing
          n114 = call <vilib>:"Trim Whitespace.vi"("string"=w289) -> ("trimmed string"=w290:string)  [unwired: 1 in]
        }
        n115 = Build Array (concatenate)(w266, w264) -> (w258:string[])
        n116 = Merge Errors(w279, w288) -> (w265:errorcluster)
        n117 = Search 1D Array(1D array=w258, element=w257) -> (index of element=w260:i32)  [unwired: 1 in]
        n118 = Greater Or Equal To 0?(x=w260) -> (x >= 0?=w261:bool)
        n119 = Select(t=w257, s=w261, f="") -> (s? t:f=w259:string)
        n120 = property on="Current Branch" class="Str"(error in=w265, "Value"=w259) -> (error out=w256:errorcluster)  [unwired: 1 in, 1 out]
        n121 = property on="Branch to Compare" class="CmbBox"(error in=w256, "Strings[]"=w258) -> (error out=w255:errorcluster, "Value"=w254:string)  [unwired: 1 in, 1 out]
        n122 = Search 1D Array(1D array=w258, element=w254) -> (index of element=w283:i32)  [unwired: 1 in]
        n123 = Greater Or Equal To 0?(x=w283) -> (x >= 0?=w282:bool)
        n124 = Select(t=w254, s=w282, f="") -> (s? t:f=w280:string)
        n125 = Bundle By Name(cluster=w285, "Branch to Compare"=w280) -> (w284:T3)
        n126 = property on="Branch to Compare" class="CmbBox"(error in=w255, "Value"=w280) -> (error out=w286:errorcluster)  [unwired: 1 in, 1 out]
      }
      frame "Stop" {
        # "Performs actions when the VI is stopped."
        n127 = for {
          tunnel: string[] ["Exit"] -> [w303] mode=indexing
          shift-right: [w305] -> w300
          shift-left: w301 -> [w306]
          shift-right: [w302] -> _
          shift-left: w299 -> [w304]
          n128 = Enqueue Element(queue=w304, element=w303, error in (no error)=w306) -> (queue out=w302:refnum<queue>, error out=w305:errorcluster)  [unwired: 1 in, 1 out]
        }
      }
      frame "Exit" {
        w309 = TRUE  # Exit?
        # "Finish the execution"
        n129 = Release Queue(queue=w308, error in (no error)=w311) -> (error out=w307:errorcluster)  [unwired: 1 in, 2 out]
      }
      frame "Error" {
        # "In case of any Git API initialization errors, we need to disable the controls."
        # "Show the error dialog and clear out the operations. Update controls status."
        n130 = call <vilib>:"Simple Error Handler.vi"("error in (no error)"=w319) -> ("error out"=w318:errorcluster)  [unwired: 4 in, 4 out]
        n131 = call <vilib>:"Clear Errors.vi"("error in (no error)"=w318) -> ("error out"=w317:errorcluster)  [unwired: 5 in, 1 out]
        n132 = Flush Queue(queue=w316, error in (no error)=w317) -> (queue out=w313:refnum<queue>, error out=w314:errorcluster)  [unwired: 1 out]
        n133 = for {
          tunnel: string[] ["Enable Disable Controls"] -> [w322] mode=indexing
          shift-right: [w324] -> w312
          shift-left: w314 -> [w325]
          shift-right: [w321] -> _
          shift-left: w313 -> [w323]
          n134 = Enqueue Element(queue=w323, element=w322, error in (no error)=w325) -> (queue out=w321:refnum<queue>, error out=w324:errorcluster)  [unwired: 1 in, 1 out]
        }
      }
    }
  }
  n135 = disable-structure shown="Enabled" {
    disable-tunnel: w4 -> [w327 w328]
    disable-tunnel: [w326 w328] -> w3
    frame Disabled {
      n136 = invoke class="VI" method="FP.Close"(error in=w327) -> (error out=w326:errorcluster)  [unwired: 2 in, 2 out]
    }
    frame Enabled {
      # "#Test"
    }
  }
  n137 = call <vilib>:"Clear Errors.vi"("error in (no error)"=w3) -> ()  [unwired: 5 in, 2 out]
